vi "driveStop.vi"(10 "reinit":bool, 11 "Velocities":cluster{"Left":dbl, "Right":dbl}) -> (2 "Done":bool, 3 "dt_outputs":cluster{"Left":dbl, "Right":dbl})   [LabVIEW 2013]
panel:
  in  "settle time":u32=250
  in  "stop deadband":dbl=1.5
  out "Waveform Chart":cluster{"Left":dbl, "Right":dbl}(graph)
  in  "max stop speed":dbl=1.5
  in  "kI":dbl=-0.008
  in  "kP":dbl=-0.1
  # "Old gains:\n\nkP -0.4\nkI -0.005\nmax stop speed 8\nstop deadband 1.5\nsettle time 250"
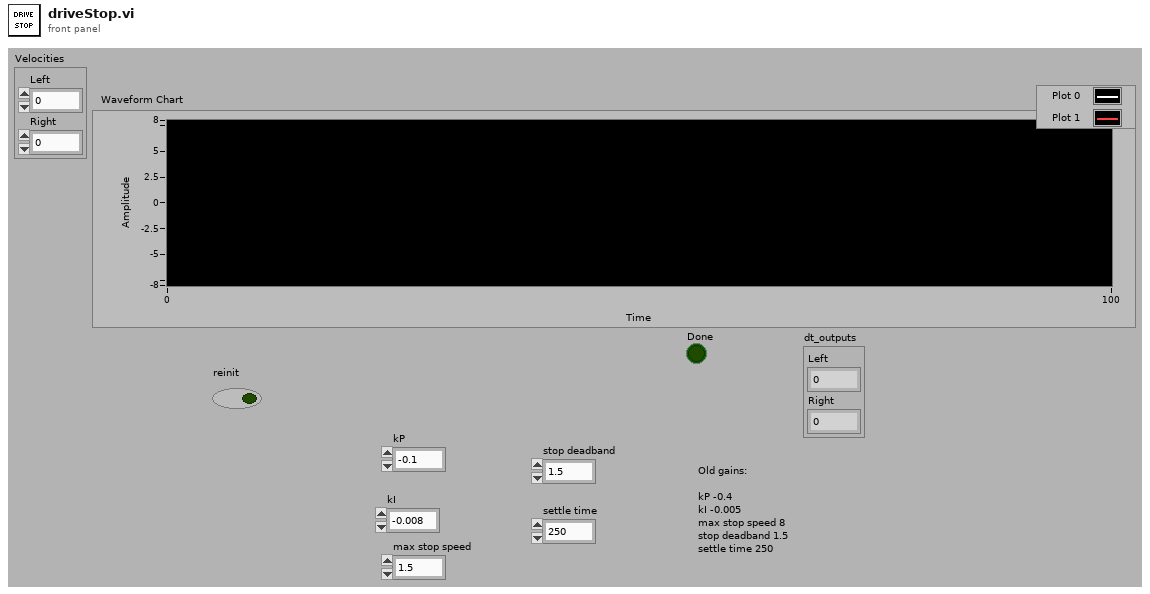
[diagram p1: front panel]
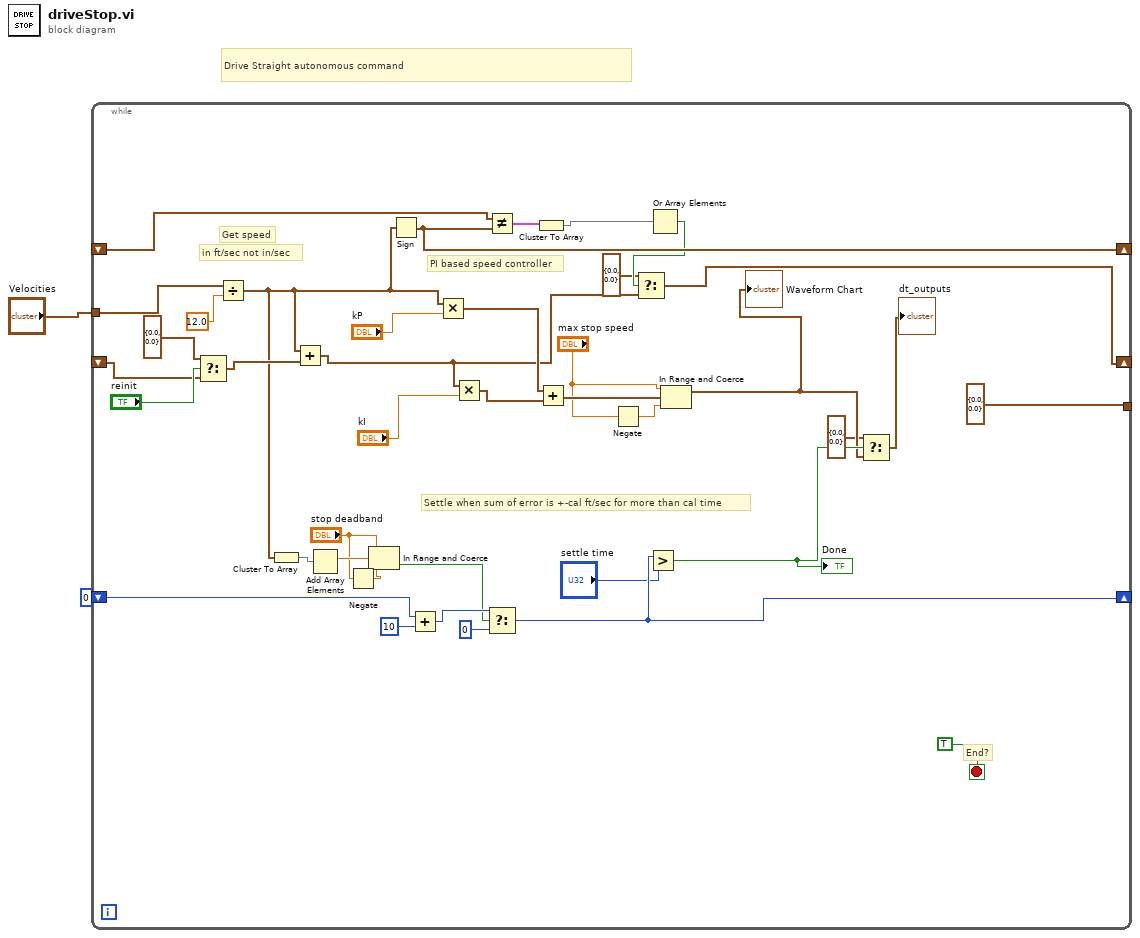
[diagram p0: block diagram]
diagram:
  # "Drive Straight autonomous command"
  n1 = while {
    tunnel: [cluster{"Left":dbl, "Right":dbl} {"Left"=0.0, "Right"=0.0} ("Drive")] -> _
    shift-right: [w6] -> _
    shift-left: _ -> [w4]
    shift-right: [w25] -> _
    shift-left: u32 0 -> [w28]
    tunnel: "Velocities" -> [w14]
    shift-right: [w11] -> _
    shift-left: _ -> [w10]
    stop <- TRUE stop-if-true
    # "Settle when sum of error is +-cal ft/sec for more than cal time"
    # "PI based speed controller"
    # "in ft/sec not in/sec"
    # "Get speed"
    # "End?"
    n2 = Select(t=cluster{"Left":dbl, "Right":dbl} {"Left"=0.0, "Right"=0.0}, s="reinit", f=w4) -> (s? t:f=w16:cluster{"Left":dbl, "Right":dbl})
    n3 = Divide(x=w14, y=12.0) -> (x/y=w12:cluster{"Left":dbl, "Right":dbl})
    n4 = Cluster To Array(cluster=w12) -> (array=w32:dbl[])
    n5 = Add(x=w12, y=w16) -> (x+y=w5:cluster{"Left":dbl, "Right":dbl})
    n6 = Add Array Elements(numeric array=w32) -> (sum=w31:dbl)
    n7 = Negate(x="stop deadband") -> (-x=w30:dbl)
    n8 = In Range and Coerce(upper limit="stop deadband", x=w31, lower limit=w30) -> (In Range?=w13:bool)  [unwired: 1 out]
    n9 = Sign(1:w12) -> (0:w11:cluster{"Left":dbl, "Right":dbl})
    n10 = Add(x=w28, y=u32 10) -> (x+y=w27:u32)
    n11 = Multiply(x=w12, y="kP") -> (x*y=w37:cluster{"Left":dbl, "Right":dbl})
    n12 = Multiply(x=w5, y="kI") -> (x*y=w36:cluster{"Left":dbl, "Right":dbl})
    n13 = Not Equal?(x=w10, y=w11) -> (x != y?=w9:cluster{"Left":bool, "Right":bool})
    n14 = Select(t=w27, s=w13, f=u32 0) -> (s? t:f=w25:u32)
    n15 = Cluster To Array(cluster=w9) -> (array=w8:bool[])
    n16 = Add(x=w37, y=w36) -> (x+y=w35:cluster{"Left":dbl, "Right":dbl})
    n17 = Negate(x="max stop speed") -> (-x=w34:dbl)
    n18 = Greater?(x=w25, y="settle time") -> (0:w21:bool)
    "Done" <- w21
    n19 = Or Array Elements(Boolean array=w8) -> (logical OR=w7:bool)
    n20 = Select(t=cluster{"Left":dbl, "Right":dbl} {"Left"=0.0, "Right"=0.0}, s=w7, f=w5) -> (s? t:f=w6:cluster{"Left":dbl, "Right":dbl})
    n21 = In Range and Coerce(upper limit="max stop speed", x=w35, lower limit=w34) -> (coerced(x)=w20:cluster{"Left":dbl, "Right":dbl})  [unwired: 1 out]
    "Waveform Chart" <- w20
    n22 = Select(t=cluster{"Left":dbl, "Right":dbl} {"Left"=0.0, "Right"=0.0}, s=w21, f=w20) -> (s? t:f=→"dt_outputs":cluster{"Left":dbl, "Right":dbl})
  }
